vi "Limit.vi"(0 "point":dbl format="%.2f", 1 "delta":dbl=1e-10 format="%.2e", 2 "formula":string) -> (3 "left limit":dbl format="%.8f", 4 "right limit":dbl format="%.8f", 5 "ticks":u32, 6 "error":i32)   [LabVIEW 2024, in "NI_Gmath.lvlib"]
doc: "<p>Determines the left and right limits of a 1D function at a given point.</p>"
uses:
  NI_Gmath.lvlib
panel:
  # "Example:\n\n point: 0.0\n delta: 1.0E-10\n formula: sin(t)/t"
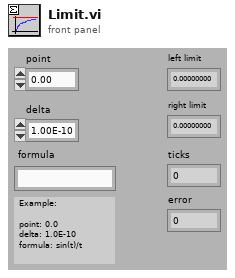
[diagram p1: front panel]
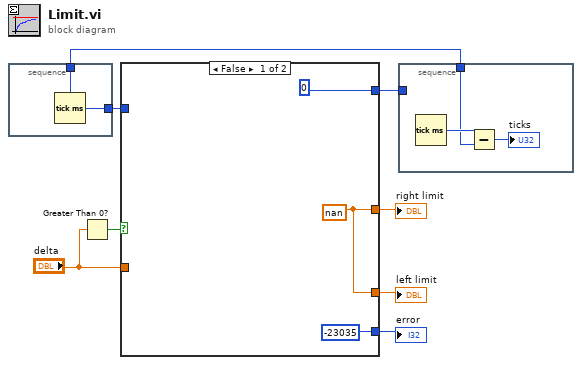
[diagram p0: block diagram]
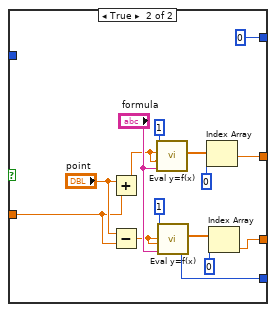
[diagram p2: hidden frame]
diagram:
  n1 = stacked-sequence {
    tunnel: [w9] -> w6
    tunnel: [w9] -> w1
    frame #0 {
      n2 = Tick Count (ms)() -> (millisecond timer value=w9:u32)
    }
  }
  n3 = Greater Than 0?(x="delta") -> (x > 0?=w3:bool)
  n4 = case shown="False" w3 {
    tunnel: [w11 w18] -> w8
    tunnel: [w11 w15] -> w7
    tunnel: [0 0] -> w5
    tunnel: "delta" -> [_ w25]
    tunnel: [-23035 w13] -> w2
    tunnel: w1 -> [_ _]
    frame False {
      w11 = nan
    }
    frame True {
      n5 = Add(x="point", y=w25) -> (x+y=w20:dbl)
      n6 = Subtract(x="point", y=w25) -> (x-y=w22:dbl)
      n7 = call "Eval y=f(x).vi"("formula"="formula", "end"=w20, "start"=w20, "number of points"=u32 1) -> ("Y Values"=w14:dbl[])  [unwired: 3 out]
      n8 = call "Eval y=f(x).vi"("formula"="formula", "end"=w22, "start"=w22, "number of points"=u32 1) -> ("error"=w13:i32, "Y Values"=w17:dbl[])  [unwired: 2 out]
      n9 = Index Array(array=w14, index=0) -> (element=w18:dbl)
      n10 = Index Array(array=w17, index=0) -> (element=w15:dbl)
    }
  }
  "right limit" <- w8
  "left limit" <- w7
  "error" <- w2
  n11 = stacked-sequence {
    tunnel: w6 -> [w28]
    tunnel: w5 -> [_]
    frame #0 {
      n12 = Tick Count (ms)() -> (millisecond timer value=w29:u32)
      n13 = Subtract(x=w29, y=w28) -> (x-y=→"ticks":u32)
    }
  }
